vi "Teleop.vi"(6 "Mode":enum16{"Tank", "Left Arcade", "Right Arcade"}(ring), 9 "Right Joystick":T1={"Device"=enum."USB 1"}, 10 "Left Joystick":T1={"Device"=enum."USB 1"}, 11 "drive.lvclass":refnum<class "drive.lvclass">) -> (3 "drive.lvclass":refnum<class "drive.lvclass">)   [LabVIEW 2015, in "drive.lvclass"]
uses:
  drive.lvclass
  <vilib>/Rock Robotics/WPI/Joystick/WPI_JoystickDevRef.ctl
  <vilib>/Rock Robotics/WPI/Joystick/WPI_JoystickDeviceEnum.ctl
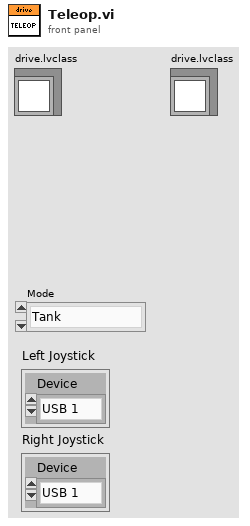
[diagram p1: front panel]
types:
  T1 = typedef "WPI_JoystickDevRef.ctl" = cluster{"Device":T2}
  T2 = typedef "WPI_JoystickDeviceEnum.ctl" = enum16{"USB 0", "USB 1", "USB 2", "USB 3", "USB 4", "USB 5"}
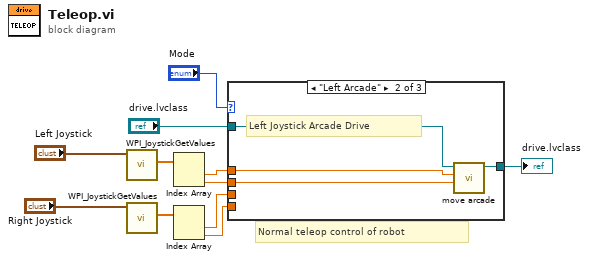
[diagram p0: block diagram]
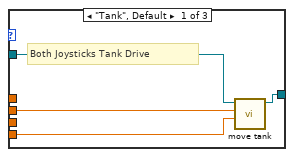
[diagram p2: hidden frame]
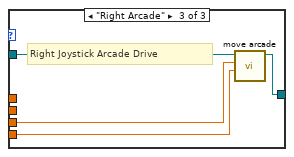
[diagram p3: hidden frame]
diagram:
  # "Normal teleop control of robot"
  n1 = call <vilib>:"WPI_JoystickGetValues.vi"("JoystickDevRef"="Left Joystick") -> ("Axes"=w7:dbl[])  [unwired: 6 in, 4 out]
  n2 = call <vilib>:"WPI_JoystickGetValues.vi"("JoystickDevRef"="Right Joystick") -> ("Axes"=w4:dbl[])  [unwired: 6 in, 4 out]
  n3 = Index Array(array=w7) -> (element #1=w6:dbl, element #2=w5:dbl)  [unwired: 2 in]
  n4 = Index Array(array=w4) -> (element #1=w2:dbl, element #2=w1:dbl)  [unwired: 2 in]
  n5 = case shown="\"Left Arcade\"" "Mode" {
    tunnel: w5 -> [w15 w19 _]
    tunnel: w1 -> [w14 _ w22]
    tunnel: w6 -> [_ w18 _]
    tunnel: w2 -> [_ _ w23]
    tunnel: "drive.lvclass" -> [w13 w17 w21]
    tunnel: [w12 w16 w20] -> w10
    frame "Tank", Default {
      # "Both Joysticks Tank Drive"
      n6 = call "move tank.vi"("Right Value"=w14, "Left Value"=w15, "drive.lvclass"=w13) -> ("drive.lvclass"=w12:refnum<class "drive.lvclass">)  [unwired: 8 in]
    }
    frame "Left Arcade" {
      # "Left Joystick Arcade Drive"
      n7 = call "move arcade.vi"("Forward Value"=w19, "Turn Value"=w18, "drive.lvclass"=w17) -> ("drive.lvclass"=w16:refnum<class "drive.lvclass">)  [unwired: 8 in]
    }
    frame "Right Arcade" {
      # "Right Joystick Arcade Drive"
      n8 = call "move arcade.vi"("Forward Value"=w22, "Turn Value"=w23, "drive.lvclass"=w21) -> ("drive.lvclass"=w20:refnum<class "drive.lvclass">)  [unwired: 8 in]
    }
  }
  "drive.lvclass" <- w10
